vi "Sequence Positions.vi"(11 "VISA resource name":refnum<visa-resource-name>="COM7") -> (2 "read string":string)   [LabVIEW 2017]
uses:
  controls/#typedef_Queue Cmd.ctl
panel:
  in  "Positions Sequence":u16[](array[slide]) max=360 step=1 scale=0.0..360.0
  in  "Exec Seq Button":bool
  in  "Callib Button":bool
  out "error out":errorcluster
  in  "error in (no error)":errorcluster
  in  "stop":bool
  in  "Get ID Button":bool
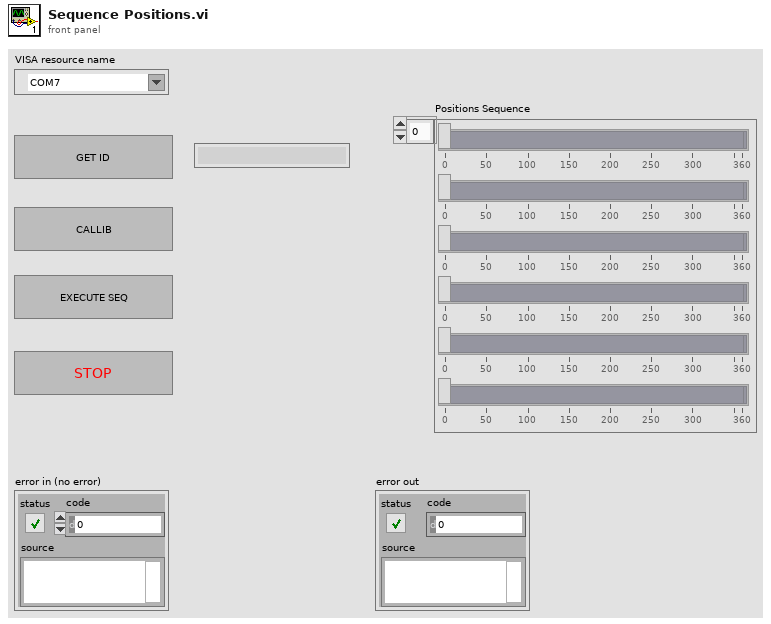
[diagram p1: front panel]
types:
  T1 = typedef "#typedef_Queue Cmd.ctl" = enum16{"Get ID", "Callib", "GoTo", "GoTo seq", "Macro seq", "Exit"}
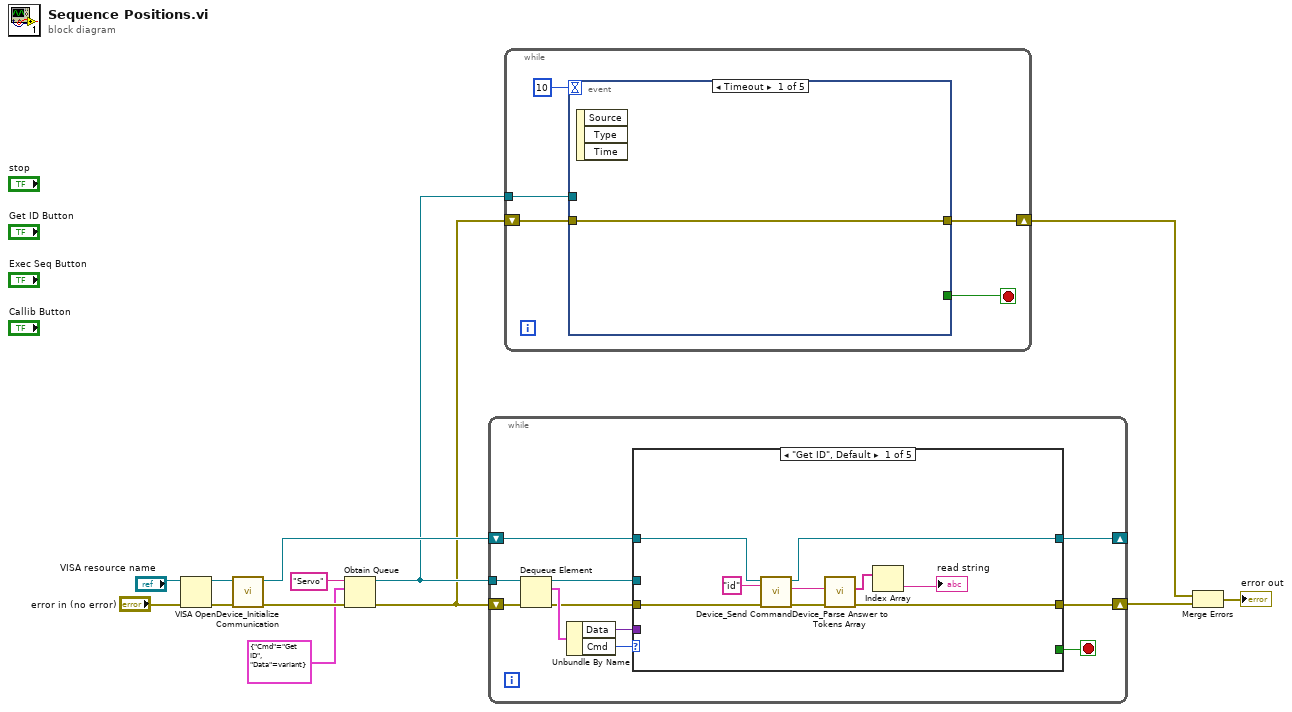
[diagram p0: block diagram]
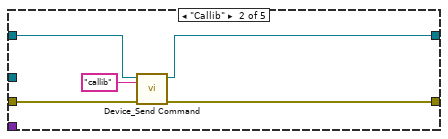
[diagram p2: hidden frame]
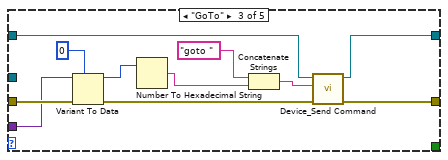
[diagram p3: hidden frame]
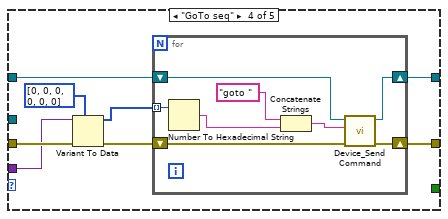
[diagram p4: hidden frame]
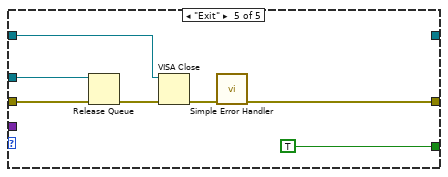
[diagram p5: hidden frame]
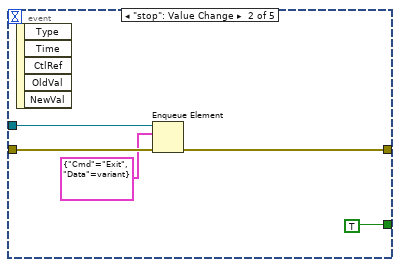
[diagram p6: hidden frame]
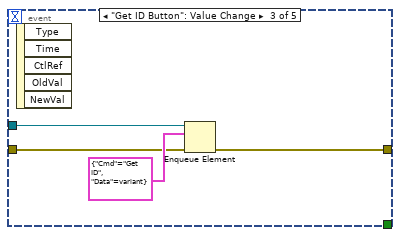
[diagram p7: hidden frame]
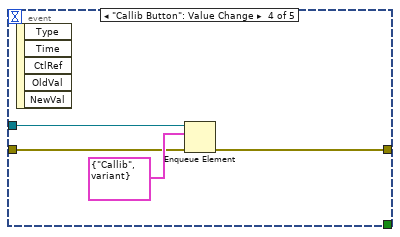
[diagram p8: hidden frame]
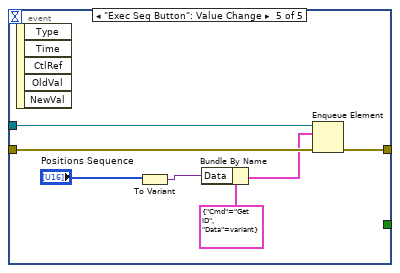
[diagram p9: hidden frame]
diagram:
  n1 = VISA Open(error in (no error)="error in (no error)", VISA resource name="VISA resource name") -> (VISA resource name=w12:refnum<visa-resource-name>, error out=w11:errorcluster)  [unwired: 3 in]
  n2 = call "Device_Initialize Communication.vi"("error in (no error)"=w11, "VISA Refnum in"=w12) -> ("error out"=w9:errorcluster, "VISA Refnum out"=w8:refnum<visa-resource-name>)  [unwired: 8 in]
  n3 = Obtain Queue(name (unnamed)="Servo", element data type=cluster{"Cmd":T1, "Data":variant} {"Cmd"=enum."Get ID", "Data"=variant} ("Queue Msg"), error in (no error)=w9) -> (queue out=w5:refnum<queue>, error out=w4:errorcluster)  [unwired: 2 in, 1 out]
  n4 = while {
    shift-right: [w15] -> _
    shift-left: w8 -> [w16]
    tunnel: w5 -> [w23]
    shift-right: [w18] -> w3
    shift-left: w4 -> [w24]
    stop <- w17 stop-if-true
    n5 = Dequeue Element(queue=w23, error in (no error)=w24) -> (queue out=w19:refnum<queue>, element=w22:cluster{"Cmd":T1, "Data":variant}, error out=w20:errorcluster)  [unwired: 1 in, 1 out]
    n6 = Unbundle By Name(w22) -> ("Data"=w14:variant, "Cmd"=w21:T1)
    n7 = case shown="\"Get ID\", Default" w21 {
      tunnel: w20 -> [w31 w36 w46 w54 w72]
      tunnel: w19 -> [_ _ _ _ w71]
      tunnel: [w28 w34 w47 w55 w66] -> w18
      tunnel: [_ _ _ _ TRUE] -> w17
      tunnel: w16 -> [w32 w37 w49 w57 w68]
      tunnel: [w30 w35 w48 w56 _] -> w15
      tunnel: w14 -> [_ _ w43 w52 _]
      frame "Get ID", Default {
        n8 = call "Device_Send Command.vi"("error in (no error)"=w31, "write string"="id", "VISA Refnum in"=w32) -> ("error out"=w29:errorcluster, "read buffer"=w27:string, "VISA Refnum out"=w30:refnum<visa-resource-name>)  [unwired: 6 in]
        n9 = call "Device_Parse Answer to Tokens Array.vi"("error in (no error)"=w29, "Answer"=w27) -> ("error out"=w28:errorcluster, "Tokens Array"=w26:string[])  [unwired: 8 in]
        n10 = Index Array(array=w26) -> (element=→"read string":string)  [unwired: 1 in]
      }
      frame "Callib" {
        n11 = call "Device_Send Command.vi"("error in (no error)"=w36, "write string"="callib", "VISA Refnum in"=w37) -> ("error out"=w34:errorcluster, "VISA Refnum out"=w35:refnum<visa-resource-name>)  [unwired: 6 in, 1 out]
      }
      frame "GoTo" {
        n12 = Variant To Data(error in=w46, type=u8 0 ("Position 2"), Variant=w43) -> (data=w42:u8, error out=w45:errorcluster)
        n13 = Number To Hexadecimal String(2:w42) -> (0:w40:string)  [unwired: 1 in]
        n14 = Concatenate Strings("goto " ("write string"), w40) -> (w39:string)
        n15 = call "Device_Send Command.vi"("error in (no error)"=w45, "write string"=w39, "VISA Refnum in"=w49) -> ("error out"=w47:errorcluster, "VISA Refnum out"=w48:refnum<visa-resource-name>)  [unwired: 6 in, 1 out]
      }
      frame "GoTo seq" {
        n16 = Variant To Data(error in=w54, type=u16[] [0, 0, 0, 0, 0, 0] ("Positions Sequence"), Variant=w52) -> (data=w50:u16[], error out=w53:errorcluster)
        n17 = for {
          shift-right: [w64] -> w56
          shift-left: w57 -> [w65]
          shift-right: [w63] -> w55
          shift-left: w53 -> [w62]
          tunnel: w50 -> [w58] mode=indexing
          n18 = Number To Hexadecimal String(2:w58) -> (0:w60:string)  [unwired: 1 in]
          n19 = Concatenate Strings("goto " ("write string"), w60) -> (w59:string)
          n20 = call "Device_Send Command.vi"("error in (no error)"=w62, "write string"=w59, "VISA Refnum in"=w65) -> ("error out"=w63:errorcluster, "VISA Refnum out"=w64:refnum<visa-resource-name>)  [unwired: 6 in, 1 out]
        }
      }
      frame "Exit" {
        n21 = Release Queue(queue=w71, error in (no error)=w72) -> (error out=w67:errorcluster)  [unwired: 1 in, 2 out]
        n22 = VISA Close(VISA resource name=w68, error in (no error)=w67) -> (error out=w69:errorcluster)
        n23 = call <vilib>:"Simple Error Handler.vi"("error in (no error)"=w69) -> ("error out"=w66:errorcluster)  [unwired: 4 in, 4 out]
      }
    }
  }
  n24 = while {
    tunnel: w5 -> [w77]
    shift-right: [w75] -> w2
    shift-left: w4 -> [w76]
    stop <- w74 stop-if-true
    n25 = event shown="[0] Timeout" {
      selector: _ -> [_ _ _ _ _]
      dyn-events: _ -> [_ _ _ _ _]
      timeout: 10 -> [_ _ _ _ _]
      tunnel: w77 -> [_ w80 w85 w89 w97]
      tunnel: w76 -> [w78 w83 w86 w90 w98]
      tunnel: [w78 w82 w84 w88 w96] -> w75
      tunnel: [_ TRUE _ _ _] -> w74
      event Timeout {
        n26 = event-data() -> ()  [unwired: 1 in, 3 out]
      }
      event "stop": Value Change {
        n27 = event-data() -> ()  [unwired: 1 in, 5 out]
        n28 = Enqueue Element(queue=w80, element=cluster{"Cmd":T1, "Data":variant} {"Cmd"=enum."Exit", "Data"=variant} ("Queue Msg"), error in (no error)=w83) -> (error out=w82:errorcluster)  [unwired: 1 in, 2 out]
      }
      event "Get ID Button": Value Change {
        n29 = event-data() -> ()  [unwired: 1 in, 5 out]
        n30 = Enqueue Element(queue=w85, element=cluster{"Cmd":T1, "Data":variant} {"Cmd"=enum."Get ID", "Data"=variant} ("Queue Msg"), error in (no error)=w86) -> (error out=w84:errorcluster)  [unwired: 1 in, 2 out]
      }
      event "Callib Button": Value Change {
        n31 = event-data() -> ()  [unwired: 1 in, 5 out]
        n32 = Enqueue Element(queue=w89, element=cluster{"Cmd":T1, "Data":variant} {"Cmd"=enum."Callib", "Data"=variant} ("Queue Msg"), error in (no error)=w90) -> (error out=w88:errorcluster)  [unwired: 1 in, 2 out]
      }
      event "Exec Seq Button": Value Change {
        n33 = event-data() -> ()  [unwired: 1 in, 5 out]
        n34 = To Variant(anything="Positions Sequence") -> (Variant=w94:variant)
        n35 = Bundle By Name(cluster=cluster{"Cmd":T1, "Data":variant} {"Cmd"=enum."Get ID", "Data"=variant} ("Queue Msg"), "Data"=w94) -> (w95:cluster{"Cmd":T1, "Data":variant})
        n36 = Enqueue Element(queue=w97, element=w95, error in (no error)=w98) -> (error out=w96:errorcluster)  [unwired: 1 in, 2 out]
      }
    }
  }
  n37 = Merge Errors(w2, w3) -> (→"error out":errorcluster)
